vi "gyro align V1.0.vi"() -> ()   [LabVIEW 2019]
uses:
  <vilib>/platform/TimedLoop/XDataNode/XDataNode.xnode
  <vilib>/Platform/TimedLoop/XDataNode/nitl_modes.ctl
  <vilib>/Platform/TimedLoop/XDataNode/XDNodeRunTimeDep.lvlib
  <vilib>/Platform/TimedLoop/XDataNode/wakeup.ctl
  <vilib>/Platform/TimedLoop/XDataNode/timing_clust.ctl
  FPGA_subVIs/low level/I2C/I2C.lvclass
panel:
  out "Waveform Chart":dbl(graph)
  in  "turn gain":dbl=1.0
  out "upper limit":dbl
  in  "stop":bool
  out "degrees out":dbl
  in  "Target angle":dbl
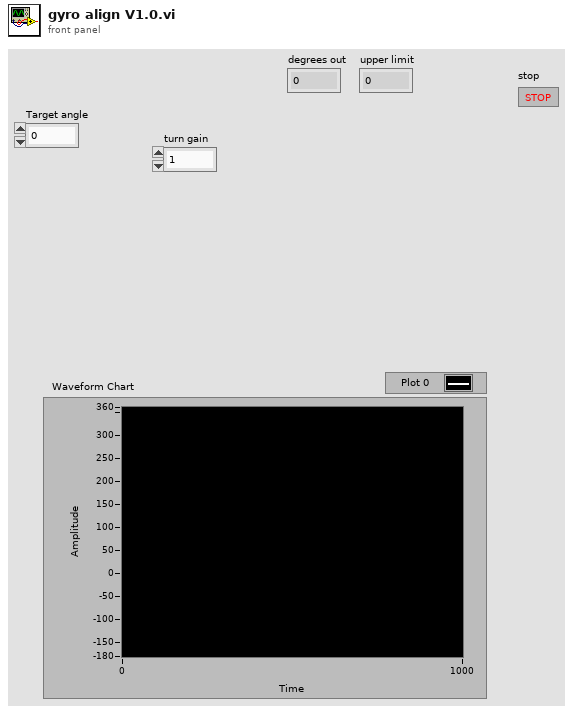
[diagram p1: front panel]
types:
  T1 = typedef "XDNodeRunTimeDep.lvlib/timing_clust.ctl" = cluster{"Expected End [f-1]":u64, "Actual End [f-1]":u64, "Finished Late? [f-1]":bool, "Expected End [i-1]":u64, "Actual End [i-1]":u64, "Finished Late? [i-1]":bool, "Expected Start [i]":u64, "Actual Start [i]":u64, "Expected Start [f]":u64, "Actual Start [f]":u64, "Source Name":string, "Structure Name":string, "Period":i64, "Deadline":i64, "Offset":i64, "Start":i64, "Priority":i32, "Timeout":i32, "Mode":T2, "Wakeup Reason":T3, "Error":errorcluster, "Source Type":string, "Secondary Source Type":string, "Global End Time":u64, "Global Start Time":u64, "Frame Duration":u64, "Iteration Duration":u64, "Assigned CPU":i32, "I/O Scan Engine Mode":u32}
  T2 = typedef "XDNodeRunTimeDep.lvlib/nitl_modes.ctl" = enum32{"No Change", "Process missed periods, maintain original phase", "Discard missed periods, maintain original phase", "Process missed periods, ignore original phase", "Discard missed periods, ignore original phase"}
  T3 = typedef "XDNodeRunTimeDep.lvlib/wakeup.ctl" = enum32{"Normal", "Aborted", "Asynchronous wakeup", "Timing source error", "Timed loop error", "Timeout"}
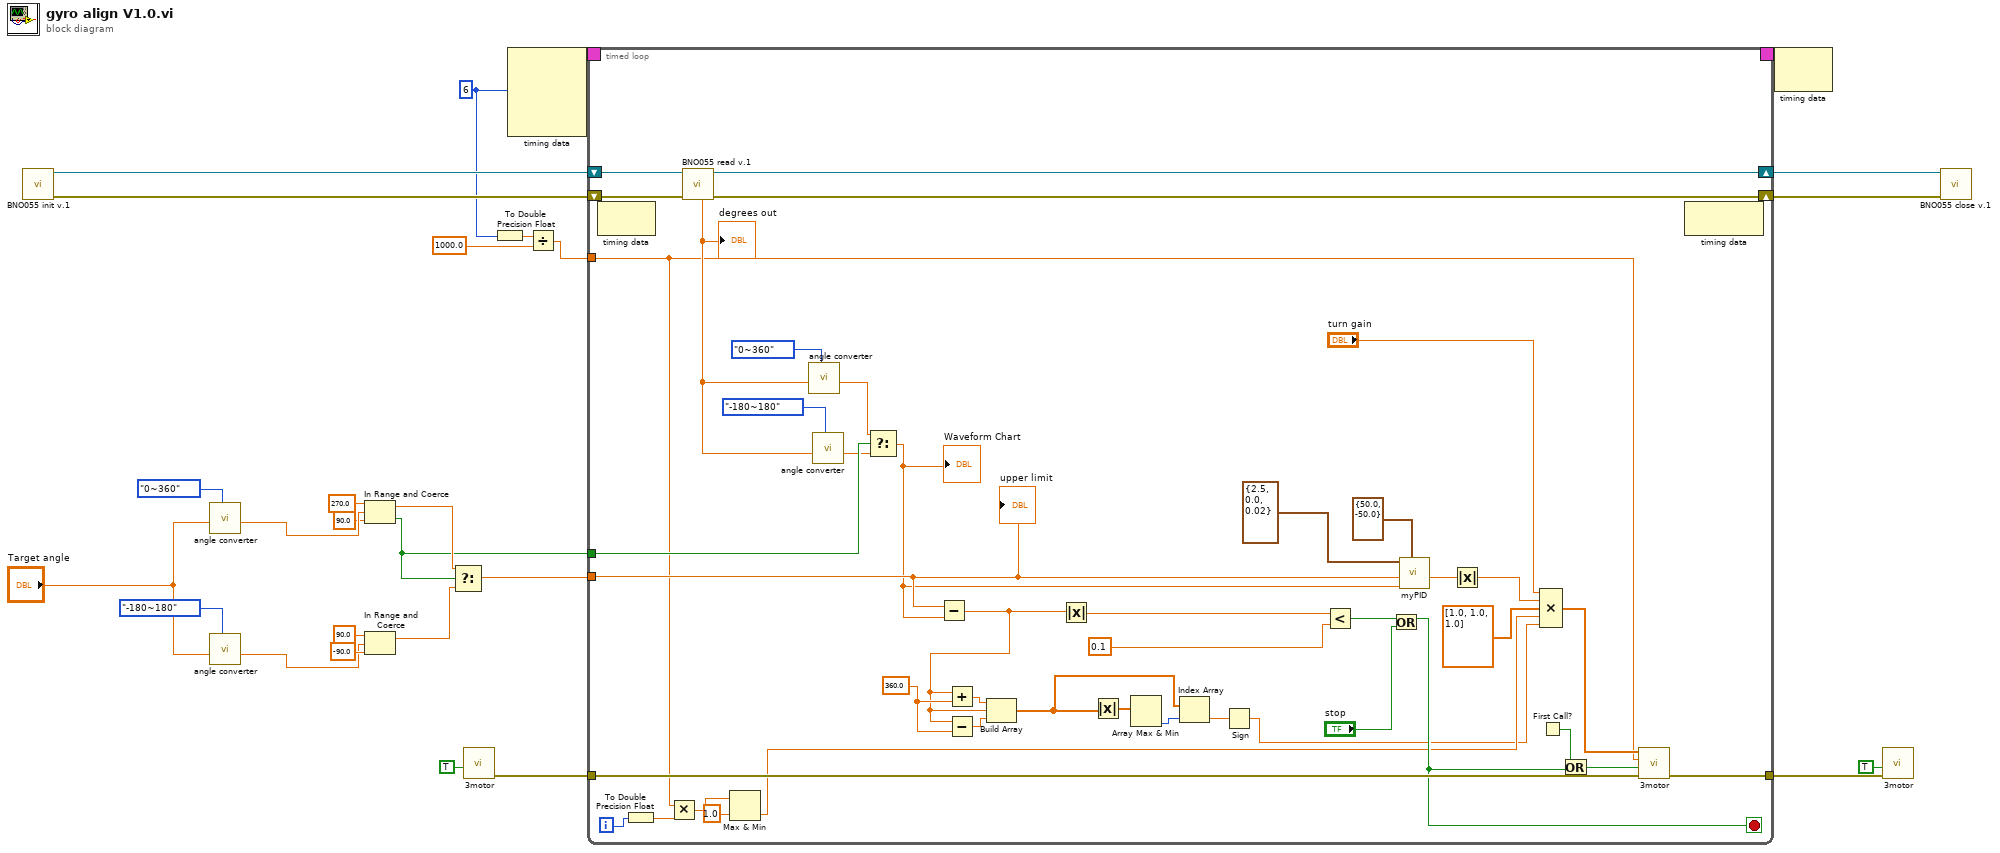
[diagram p0: block diagram]
diagram:
  w6 = i64 6 ("Period")
  n1 = call "BNO055 init v.1.vi"() -> ("error out"=w15:errorcluster, "I2C out"=w14:refnum<class "I2C.lvclass">)  [unwired: 10 in]
  n2 = call "angle converter.vi"("select"=enum16{"-180~180", "0~360"}."0~360", "input angle"="Target angle") -> ("angle out"=w22:dbl)  [unwired: 9 in]
  n3 = call "angle converter.vi"("select"=enum16{"-180~180", "0~360"}."-180~180", "input angle"="Target angle") -> ("angle out"=w25:dbl)  [unwired: 9 in]
  n4 = In Range and Coerce(upper limit=270.0, x=w22, lower limit=90.0) -> (coerced(x)=w18:dbl, In Range?=w16:bool)
  n5 = In Range and Coerce(upper limit=90.0, x=w25, lower limit=-90.0) -> (coerced(x)=w17:dbl)  [unwired: 1 out]
  n6 = Select(t=w18, s=w16, f=w17) -> (s? t:f=w11:dbl)
  n7 = call "3motor.vi"("Reset"=TRUE) -> ("error out"=w7:errorcluster)  [unwired: 9 in, 1 out]
  n8 = To Double Precision Float(number=w6) -> (double precision float=w5:dbl)
  n9 = node-c288(w6) -> (w10:T1)  [unwired: 3 in]
  n10 = Divide(x=w5, y=1000.0) -> (x/y=w3:dbl)
  n11 = timed-loop {
    timing: w10 -> [_]
    timing-out: [_] -> w9
    tunnel: w16 -> [w68]
    tunnel: w11 -> [w49]
    shift-right: [w64] -> w13
    shift-left: w15 -> [w67]
    shift-right: [w63] -> w12
    shift-left: w14 -> [w66]
    tunnel: w7 -> [w58]
    tunnel: w3 -> [w44]
    tunnel: [w54] -> w2
    i -> [w46]
    stop <- w51 stop-if-true
    w38 = 360.0
    n12 = node-c288() -> ()  [unwired: 1 in, 1 out]
    n13 = To Double Precision Float(number=w46) -> (double precision float=w45:dbl)
    n14 = Multiply(x=w44, y=w45) -> (x*y=w43:dbl)
    n15 = call "BNO055 read v.1.vi"("error in (no error)"=w67, "I2C in"=w66) -> ("error out"=w64:errorcluster, "I2C out"=w63:refnum<class "I2C.lvclass">, "yaw"=w65:dbl)  [unwired: 5 in, 2 out]
    "degrees out" <- w65
    n16 = Max & Min(x=w43, y=1.0) -> (min(x,y)=w41:dbl)  [unwired: 1 out]
    n17 = call "angle converter.vi"("select"=enum16{"-180~180", "0~360"}."0~360", "input angle"=w65) -> ("angle out"=w53:dbl)  [unwired: 9 in]
    n18 = call "angle converter.vi"("select"=enum16{"-180~180", "0~360"}."-180~180", "input angle"=w65) -> ("angle out"=w52:dbl)  [unwired: 9 in]
    n19 = Select(t=w53, s=w68, f=w52) -> (s? t:f=w28:dbl)
    "Waveform Chart" <- w28
    n20 = Subtract(x=w49, y=w28) -> (x-y=w32:dbl)
    n21 = Add(x=w32, y=w38) -> (x+y=w37:dbl)
    n22 = Subtract(x=w32, y=w38) -> (x-y=w36:dbl)
    n23 = Build Array(w37, w32, w36) -> (w33:dbl[])
    n24 = Absolute Value(x=w32) -> (abs(x)=w40:dbl)
    n25 = Absolute Value(x=w33) -> (abs(x)=w35:dbl[])
    n26 = Array Max & Min(array=w35) -> (min index (indices)=w34:i32)  [unwired: 3 out]
    n27 = Index Array(array=w33, index=w34) -> (element=w31:dbl)
    n28 = Sign(1:w31) -> (0:w39:dbl)
    n29 = Less?(x=w40, y=0.1) -> (x < y?=w48:bool)
    n30 = Or(x=w48, y="stop") -> (x .or. y?=w51:bool)
    n31 = call "myPID.vi"("output range"=cluster{"output high":dbl, "output low":dbl} {"output high"=50.0, "output low"=-50.0}, "Processer"=w28, "setpoint"=w49, "PID"=cluster{"Kp":dbl, "Ki":dbl, "Kd":dbl} {"Kp"=2.5, "Ki"=0.0, "Kd"=0.02}) -> ("out"=w60:dbl)  [unwired: 6 in, 1 out]
    n32 = Absolute Value(x=w60) -> (abs(x)=w29:dbl)
    n33 = First Call?() -> (First Call?: T/F=w56:bool)
    n34 = Compound Arithmetic op=MULTIPLY("turn gain", w29, dbl[] [1.0, 1.0, 1.0], w41, w39) -> (w55:dbl[])
    n35 = Or(x=w56, y=w51) -> (x .or. y?=w57:bool)
    n36 = call "3motor.vi"("error in (no error)"=w58, "Reset"=w57, "dt(s)"=w44, "Motor speed"=w55) -> ("error out"=w54:errorcluster)  [unwired: 6 in, 1 out]
    n37 = node-c288() -> ()  [unwired: 1 in, 1 out]
    "upper limit" <- w49
  }
  n38 = node-c288(w9) -> ()  [unwired: 1 out]
  n39 = call "3motor.vi"("error in (no error)"=w2, "Reset"=TRUE) -> ()  [unwired: 8 in, 2 out]
  n40 = call "BNO055 close v.1.vi"("error in (no error)"=w13, "I2C Ref In"=w12) -> ()  [unwired: 9 in, 1 out]
